vi "updateTemplateForNewCSC.vi"() -> ()   [LabVIEW 2016]
uses:
  Typedefs/LibraryDirectories.ctl
  Typedefs/LibraryMemberNameReplacement.ctl
  <vilib>/Utility/miscctls.llb/LVPointTypeDef.ctl
panel:
  out "Array 3":path[](array[path])
  out "Array 2":string[](array[string])
  out "Array":string[](array[string])
  out "VI Name":string
  out "error out":errorcluster
  in  "Subprojects directory":path=path "/home/plotz/lsst_ts/ts_AtSpectrograph/Subprojects"
  in  "New CSC Name":string="AtSpectrograph"
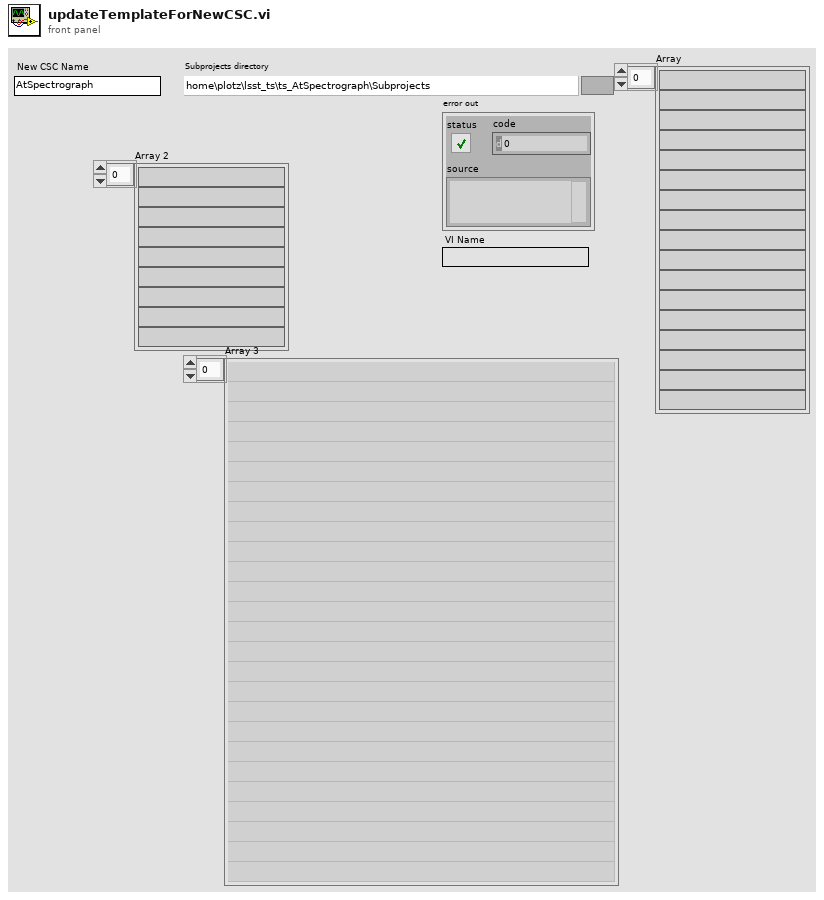
[diagram p1: front panel]
types:
  T1 = typedef "LibraryMemberNameReplacement.ctl" = cluster{"String To Replace in VI names":string, "String To Replace in Control names":string, "New String in VI names":string, "New String in Control names":string}
  T2 = typedef "LibraryDirectories.ctl" = cluster{"OldLibraryDirectory":string, "NewLibraryDirectory":string}
  T3 = cluster{"OldLibrary":string, "NewLibrary":string}
  T4 = typedef "LVPointTypeDef.ctl" = cluster{"Horizontal":i16, "Vertical":i16}
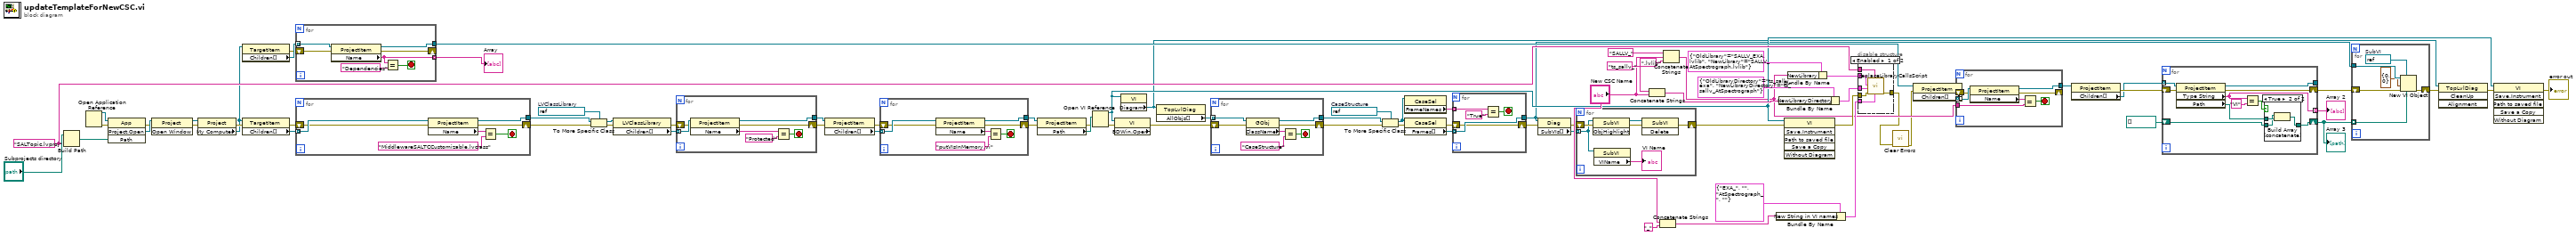
[diagram p0: block diagram]
diagram:
  w38 = refnum<vi> refnum  # CaseStructure
  w57 = refnum<vi> refnum  # LVClassLibrary
  w65 = "SALTopic.lvproj" ("name or relative path")
  n1 = Build Path(base path="Subprojects directory", name or relative path=w65) -> (appended path=w63:path)
  n2 = Open Application Reference() -> (0:w62:errorcluster, 3:w64:refnum<vi>)  [unwired: 4 in]
  n3 = invoke class="App" method="Project.Open"(reference=w64, error in=w62, "Path"=w63) -> (error out=w52:errorcluster, "Project:Open"=w61:refnum<vi>)  [unwired: 1 in, 2 out]
  n4 = invoke class="Project" method="Open Window"(reference=w61, error in=w52) -> (reference out=w60:refnum<vi>, error out=w53:errorcluster)  [unwired: 1 in, 1 out]
  n5 = property class="Project"(reference=w60, error in=w53) -> (error out=w51:errorcluster, "My Computer"=w22:refnum<vi>)  [unwired: 1 out]
  n6 = property class="TargetItem"(reference=w22) -> (error out=w23:errorcluster, "Children[]"=w24:refnum<vi>[])  [unwired: 1 in, 1 out]
  n7 = property class="TargetItem"(reference=w22, error in=w51) -> (error out=w50:errorcluster, "Children[]"=w59:refnum<vi>[])  [unwired: 1 out]
  n8 = for {
    tunnel: w24 -> [w86] mode=indexing
    tunnel: [w83] -> w20
    shift-right: [w81] -> _
    shift-left: w23 -> [w82]
    tunnel: [w80] -> w21 mode=indexing
    stop <- w84 stop-if-true
    n9 = property class="ProjectItem"(reference=w86, error in=w82) -> (reference out=w83:refnum<vi>, error out=w81:errorcluster, "Name"=w80:string)
    n10 = Equal?(x=w80, y="Dependencies") -> (x = y?=w84:bool)
  }
  "Array" <- w21
  n11 = for {
    tunnel: w59 -> [w93] mode=indexing
    tunnel: [w89] -> w58
    shift-right: [w87] -> w49
    shift-left: w50 -> [w88]
    stop <- w90 stop-if-true
    n12 = property class="ProjectItem"(reference=w93, error in=w88) -> (reference out=w89:refnum<vi>, error out=w87:errorcluster, "Name"=w92:string)
    n13 = Equal?(x=w92, y="MiddlewareSALTCCustomizable.lvclass") -> (x = y?=w90:bool)
  }
  n14 = To More Specific Class(target class=w57, reference=w58, error in=w49) -> (specific class reference=w56:refnum<vi>, error out=w48:errorcluster)
  n15 = property class="LVClassLibrary"(reference=w56, error in=w48) -> (error out=w18:errorcluster, "Children[]"=w44:refnum<vi>[])  [unwired: 1 out]
  n16 = for {
    tunnel: w44 -> [w100] mode=indexing
    tunnel: [w96] -> w45
    shift-right: [w95] -> w43
    shift-left: w18 -> [w94]
    stop <- w97 stop-if-true
    n17 = property class="ProjectItem"(reference=w100, error in=w94) -> (reference out=w96:refnum<vi>, error out=w95:errorcluster, "Name"=w99:string)
    n18 = Equal?(x=w99, y="Protected") -> (x = y?=w97:bool)
  }
  n19 = property class="ProjectItem"(reference=w45, error in=w43) -> (error out=w39:errorcluster, "Children[]"=w42:refnum<vi>[])  [unwired: 1 out]
  n20 = for {
    tunnel: w42 -> [w107] mode=indexing
    tunnel: [w103] -> w55
    shift-right: [w102] -> w47
    shift-left: w39 -> [w101]
    stop <- w104 stop-if-true
    n21 = property class="ProjectItem"(reference=w107, error in=w101) -> (reference out=w103:refnum<vi>, error out=w102:errorcluster, "Name"=w106:string)
    n22 = Equal?(x=w106, y="putVIsInMemory.vi") -> (x = y?=w104:bool)
  }
  n23 = property class="ProjectItem"(reference=w55, error in=w47) -> (error out=w46:errorcluster, "Path"=w54:path)  [unwired: 1 out]
  n24 = Open VI Reference(vi path=w54, error in (no error)=w46) -> (vi reference=w9:refnum<vi>, error out=w41:errorcluster)  [unwired: 4 in]
  n25 = property class="VI" props=["BDWin.Open"](reference=w9, error in=w41) -> (error out=w34:errorcluster)  [unwired: 2 out]
  n26 = property class="VI"(reference=w9) -> ("Diagram"=w5:refnum<vi>)  [unwired: 1 in, 2 out]
  n27 = property class="TopLvlDiag"(reference=w5) -> ("AllObjs[]"=w40:refnum<vi>[])  [unwired: 1 in, 2 out]
  n28 = for {
    tunnel: w40 -> [w114] mode=indexing
    tunnel: [w110] -> w37
    shift-right: [w109] -> w36
    shift-left: w34 -> [w108]
    stop <- w111 stop-if-true
    n29 = property class="GObj"(reference=w114, error in=w108) -> (reference out=w110:refnum<vi>, error out=w109:errorcluster, "ClassName"=w113:string)
    n30 = Equal?(x=w113, y="CaseStructure") -> (x = y?=w111:bool)
  }
  n31 = To More Specific Class(target class=w38, reference=w37, error in=w36) -> (specific class reference=w28:refnum<vi>, error out=w32:errorcluster)
  n32 = property class="CaseSel"(reference=w28) -> ("FrameNames"=w27:string[])  [unwired: 1 in, 2 out]
  n33 = property class="CaseSel"(reference=w28, error in=w32) -> (error out=w33:errorcluster, "Frames[]"=w35:refnum<vi>[])  [unwired: 1 out]
  n34 = for {
    tunnel: w35 -> [w119] mode=indexing
    tunnel: [w119] -> w6
    shift-right: [w116] -> w30
    shift-left: w33 -> [w116]
    tunnel: w27 -> [w118] mode=indexing
    stop <- w115 stop-if-true
    n35 = Equal?(x=w118, y="True") -> (x = y?=w115:bool)
  }
  n36 = property class="Diag"(reference=w6, error in=w30) -> (error out=w29:errorcluster, "SubVIs[]"=w31:refnum<vi>[])  [unwired: 1 out]
  n37 = for {
    tunnel: w31 -> [w124] mode=indexing
    shift-right: [w121] -> w26
    shift-left: w29 -> [w125]
    n38 = invoke class="SubVI" method="ObjHighlight"(reference=w124, error in=w125) -> (reference out=w123:refnum<vi>, error out=w122:errorcluster)  [unwired: 1 in, 1 out]
    n39 = property class="SubVI"(reference=w124) -> ("VIName"=→"VI Name":string)  [unwired: 1 in, 2 out]
    n40 = invoke class="SubVI" method="Delete"(reference=w123, error in=w122) -> (error out=w121:errorcluster)  [unwired: 1 in, 2 out]
  }
  n41 = Concatenate Strings("ts_sallv_" ("string"), "New CSC Name") -> (w73:string)
  n42 = Concatenate Strings("New CSC Name", "_" ("string")) -> (w68:string)
  n43 = Concatenate Strings("SALLV_" ("string"), "New CSC Name", ".lvlib" ("string")) -> (w4:string)
  n44 = Bundle By Name(cluster=T1 {"String To Replace in VI names"="EXA_", "String To Replace in Control names"="", "New String in VI names"="AtSpectrograph_", "New String in Control names"=""} ("Library Member Name Replacement"), "New String in VI names"=w68) -> (w67:T1)
  n45 = Bundle By Name(cluster=T2 {"OldLibraryDirectory"="ts_sallv_exa", "NewLibraryDirectory"="ts_sallv_AtSpectrograph"} ("LibraryDirectories"), "NewLibraryDirectory"=w73) -> (w72:T2)
  n46 = invoke class="VI" method="Save.Instrument"(reference=w9, error in=w26) -> (error out=w25:errorcluster)  [unwired: 4 in, 5 out]
  n47 = Bundle By Name(cluster=T3 {"OldLibrary"="SALLV_EXA.lvlib", "NewLibrary"="SALLV_AtSpectrograph.lvlib"} ("Libraries"), "NewLibrary"=w4) -> (w76:T3)
  n48 = disable-structure shown="Enabled" {
    disable-tunnel: w76 -> [w131 _]
    disable-tunnel: w72 -> [w130 _]
    disable-tunnel: w67 -> [w129 _]
    disable-tunnel: w65 -> [w128 _]
    disable-tunnel: [w127 _] -> w2
    disable-tunnel: w25 -> [w126 _]
    frame Enabled {
      n49 = call "replaceLibraryCallsScript.vi"("Library Member Name Replacement"=w129, "Project To Modify"=w128, "error in (no error)"=w126, "LibraryDirectories"=w130, "Libraries"=w131) -> ("error out"=w127:errorcluster)  [unwired: 6 in]
    }
    frame Disabled {
    }
  }
  n50 = call <vilib>:"Clear Errors.vi"("error in (no error)"=w2) -> ("error out"=w1:errorcluster)  [unwired: 5 in, 1 out]
  n51 = property class="ProjectItem"(reference=w20, error in=w1) -> (error out=w17:errorcluster, "Children[]"=w19:refnum<vi>[])  [unwired: 1 out]
  n52 = for {
    tunnel: w19 -> [w138] mode=indexing
    tunnel: [w135] -> w14
    shift-right: [w134] -> _
    shift-left: w17 -> [w133]
    tunnel: w4 -> [w132]
    stop <- w136 stop-if-true
    n53 = property class="ProjectItem"(reference=w138, error in=w133) -> (reference out=w135:refnum<vi>, error out=w134:errorcluster, "Name"=w137:string)
    n54 = Equal?(x=w137, y=w132) -> (x = y?=w136:bool)
  }
  n55 = property class="ProjectItem"(reference=w14) -> (error out=w16:errorcluster, "Children[]"=w15:refnum<vi>[])  [unwired: 1 in, 1 out]
  n56 = for {
    tunnel: w15 -> [w148] mode=indexing
    tunnel: [w146] -> _
    shift-right: [w145] -> w3
    shift-left: w16 -> [w144]
    tunnel: [w143] -> w13 mode=indexing
    shift-right: [w141] -> w11
    shift-left: path[] [] -> [w140]
    n57 = property class="ProjectItem"(reference=w148, error in=w144) -> (reference out=w146:refnum<vi>, error out=w145:errorcluster, "Type String"=w143:string, "Path"=w142:path)
    n58 = Equal?(x=w143, y="VI") -> (x = y?=w139:bool)
    n59 = case shown="True" w139 {
      tunnel: w142 -> [_ w152]
      tunnel: [w149 w151] -> w141
      tunnel: w140 -> [w149 w150]
      frame False {
      }
      frame True {
        n60 = Build Array (concatenate)(w150, w152) -> (w151:path[])
      }
    }
  }
  "Array 2" <- w13
  "Array 3" <- w11
  n61 = for {
    tunnel: w6 -> [w158]
    tunnel: w11 -> [w157] mode=indexing
    shift-right: [w154] -> w8
    shift-left: w3 -> [w155]
    w156 = refnum<vi> refnum  # SubVI
    n62 = New VI Object(vi object class=w156, owner refnum=w158, position/next to=T4 {"Horizontal"=0, "Vertical"=0} ("location"), 6:w157, 8:w155) -> (0:w154:errorcluster)  [unwired: 3 in, 1 out]
  }
  n63 = invoke class="TopLvlDiag" method="CleanUp"(reference=w5, error in=w8) -> (error out=w7:errorcluster)  [unwired: 2 in, 3 out]
  n64 = invoke class="VI" method="Save.Instrument"(reference=w9, error in=w7) -> (error out=→"error out":errorcluster)  [unwired: 4 in, 5 out]
